vi "Periodic Tasks.vi"(8 "error in":errorcluster) -> ()   [LabVIEW 2018]
doc: "This VI runs in parallel to other tasks. It can contain as many user-defined periodic loops as you need. These can carry out PID or other sorts of timed response."
uses:
  SwerveRotationCalibrate.ctl
  <vilib>/Rock Robotics/WPI/ThirdParty/Phoenix-LabVIEW/Motor Controller/Controls/CTRE_Phoenix_MotorControl_NeutralMode.ctl
  <vilib>/Rock Robotics/WPI/ThirdParty/Phoenix-LabVIEW/Motor Controller/Controls/CTRE_Phoenix_MotorControl_ControlMode.ctl
  <vilib>/Rock Robotics/WPI/ThirdParty/Phoenix-LabVIEW/Motor Controller/Controls/CTRE_Phoenix_MotorControl_FeedbackDevice.ctl
  HatchModes.ctl
  ElevBasePos.ctl
  ElevModes.ctl
  SequenceActions.ctl
  d8969dce-e83f-414b-ab1b-b6caec8a5545.vi
  a102eae3-c5ed-494b-96cc-72fbbd712b4d.vi
  <vilib>/Rock Robotics/WPI/Utilities/WPI_GetSetVariantRefNum.vi
  <vilib>/Rock Robotics/Network Tables/NT Read Boolean.vi
  Robot Global Data.vi
  <vilib>/Rock Robotics/Network Tables/NT Write Numeric Array.vi
  <vilib>/Rock Robotics/Network Tables/NT Write String.vi
  <vilib>/Rock Robotics/Network Tables/NT Write Number.vi
  <vilib>/Rock Robotics/Network Tables/NT Write Boolean.vi
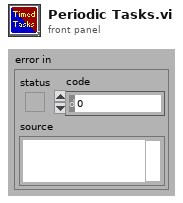
[diagram p1: front panel]
types:
  T1 = typedef "HatchModes.ctl" = enum16{"Travel", "PickPlace"}
  T2 = typedef "SwerveRotationCalibrate.ctl" = enum16{"Calibrate", "Home", "ManualHome", "ResetQuad", "Drive"}
  T3 = typedef "CTRE_Phoenix_MotorControl_NeutralMode.ctl" = enum8{"EEPROMSetting", "Override to Coast", "Override to Brake"}
  T4 = typedef "CTRE_Phoenix_MotorControl_ControlMode.ctl" = u16
  T5 = typedef "CTRE_Phoenix_MotorControl_FeedbackDevice.ctl" = i8
  T6 = cluster{"T0":u32, "Mode":T2, "Rotation Neutral Mode":T3, "Rotation Control Mode":T4, "Feedback Device":T5}
  T7 = cluster{"Yaw":dbl, "Roll":dbl, "Pitch":dbl, "Heading":dbl, "Fused Heading":dbl}
  T8 = typedef "ElevBasePos.ctl" = enum16{"NoChange", "Hatch", "Unused", "Carry", "Cargo"}
  T9 = typedef "WPI_JoystickDevRef.ctl" = cluster{"Device":T10}
  T10 = typedef "WPI_JoystickDeviceEnum.ctl" = enum16{"USB 0", "USB 1", "USB 2", "USB 3", "USB 4", "USB 5"}
  T11 = typedef "ElevModes.ctl" = enum16{"Manual", "Auto"}
  T12 = typedef "SequenceActions.ctl" = enum16{"HatchLatch", "MoveElev", "Ready"}
  T13 = typedef "WPI_DriverStationRobotMode2.ctl" = enum16{"Autonomous Disabled", "Autonomous Enabled", "Teleop Disabled", "Teleop Enabled", "Disconnected", "Finish", "Test Disabled", "Test Enabled", "Emergency Stopped"}
  T14 = cluster{"Buttons[0]":bool, "Buttons[1]":bool, "Buttons[2]":bool, "Buttons[3]":bool, "Buttons[4]":bool, "Buttons[5]":bool, "Buttons[6]":bool, "Buttons[7]":bool, "Buttons[8]":bool, "Buttons[9]":bool, "Buttons[10]":bool, "Buttons[11]":bool, "Buttons[12]":bool}
  T15 = cluster{"Motor1":cluster{"P":dbl, "I":dbl, "D":dbl}, "Motor3":cluster{"P":dbl, "I":dbl, "D":dbl}, "Motor2":cluster{"P":dbl, "I":dbl, "D":dbl}, "Motor4":cluster{"P":dbl, "I":dbl, "D":dbl}}
  T16 = typedef "WPI_CompressorDevRef.ctl" = cluster{"DevStatus":errorcluster, "Pneumatics Control Module":u8}
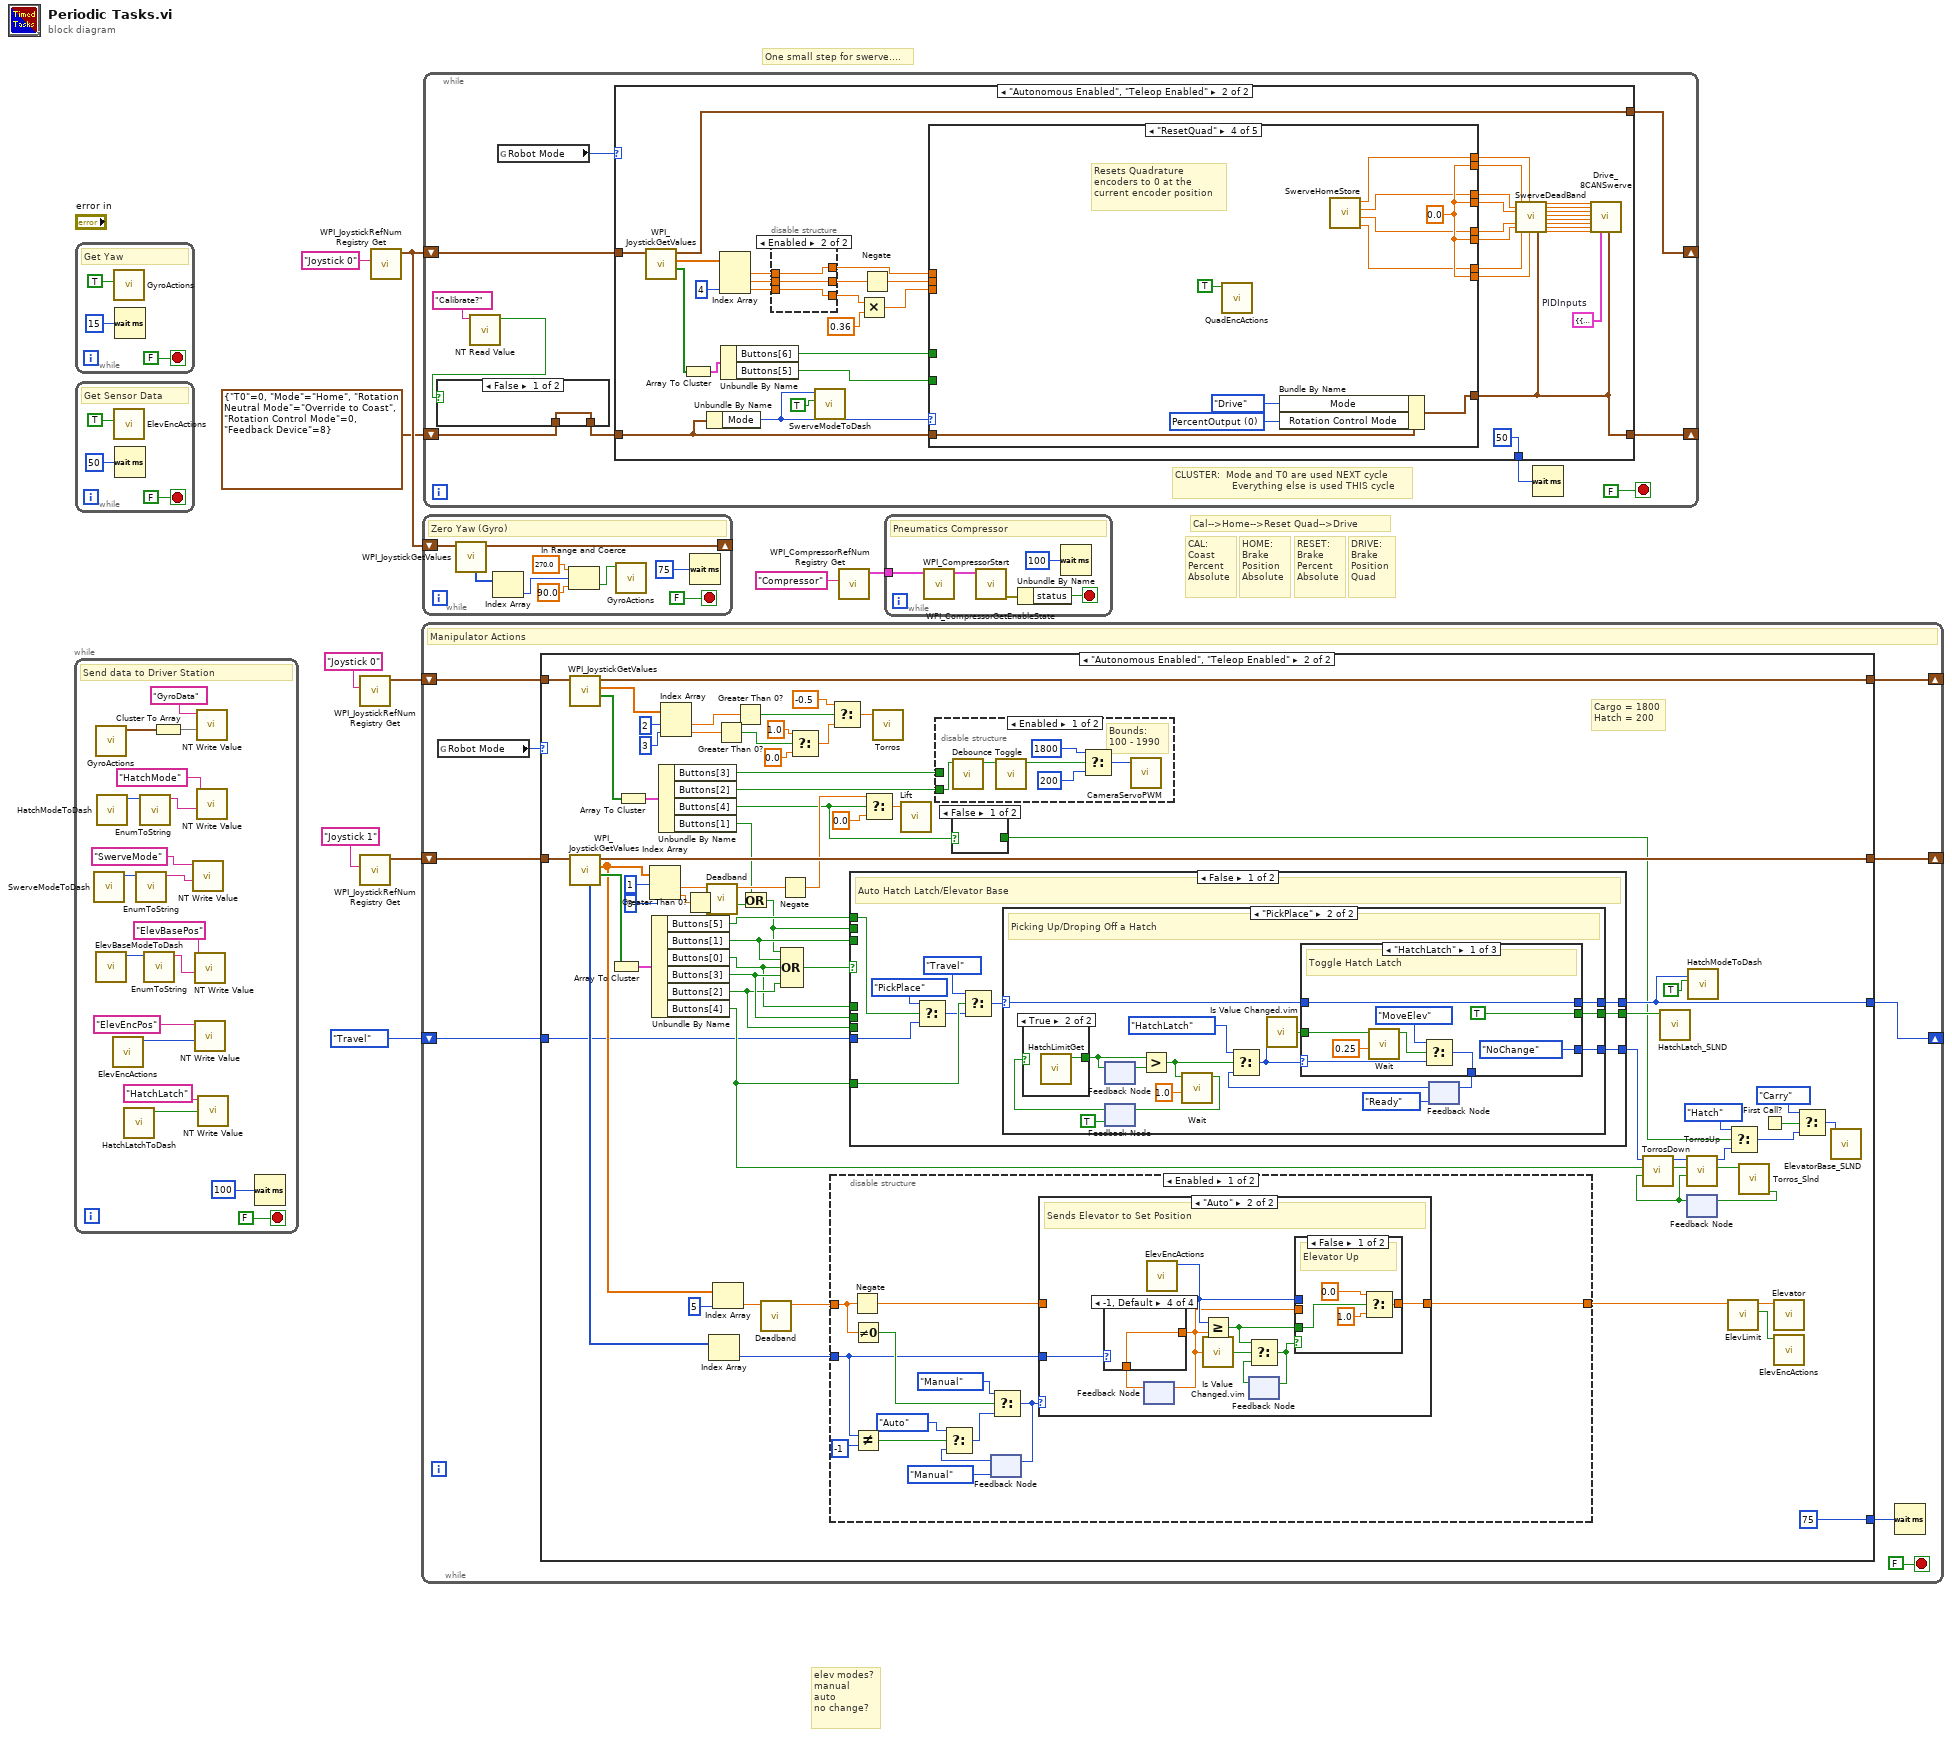
[diagram p0: block diagram]
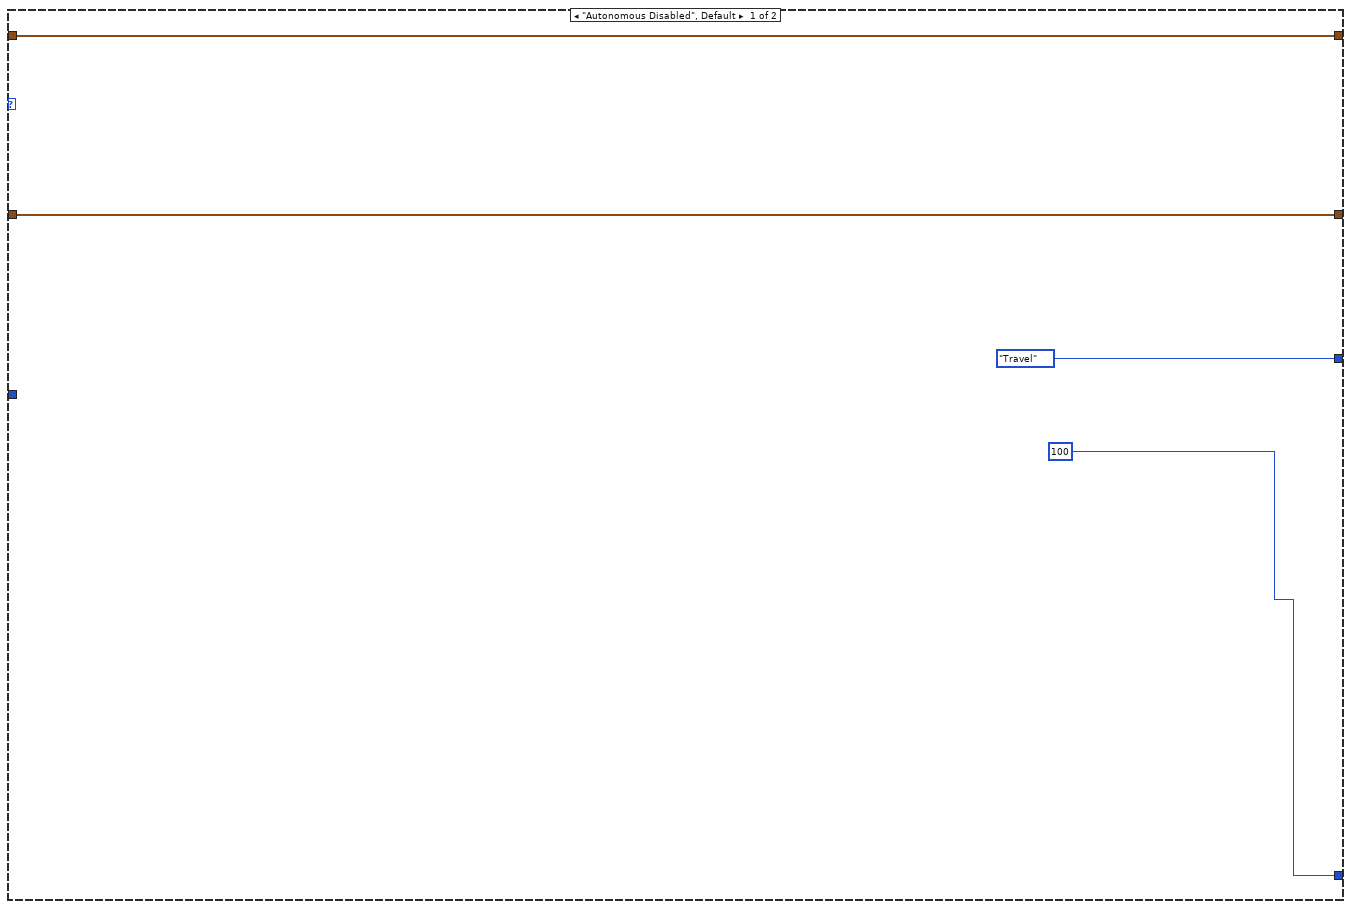
[diagram p2: hidden frame]
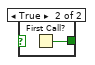
[diagram p3: hidden frame]
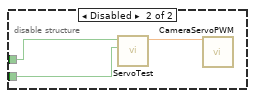
[diagram p4: hidden frame]
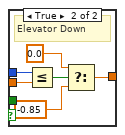
[diagram p6: hidden frame]
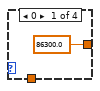
[diagram p7: hidden frame]
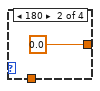
[diagram p8: hidden frame]
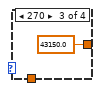
[diagram p9: hidden frame]
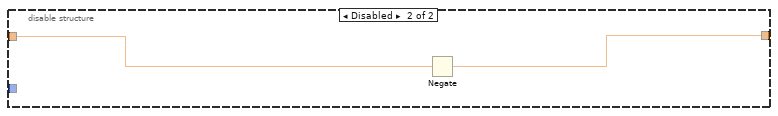
[diagram p10: hidden frame]
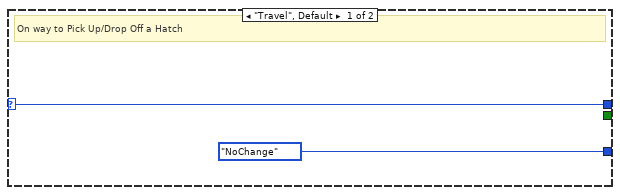
[diagram p11: hidden frame]
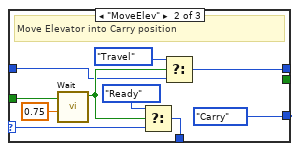
[diagram p13: hidden frame]
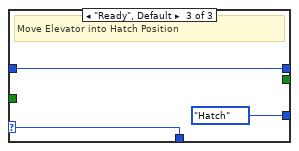
[diagram p14: hidden frame]
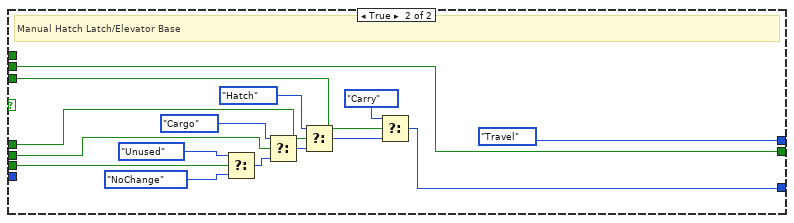
[diagram p15: hidden frame]
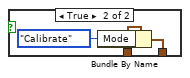
[diagram p16: hidden frame]
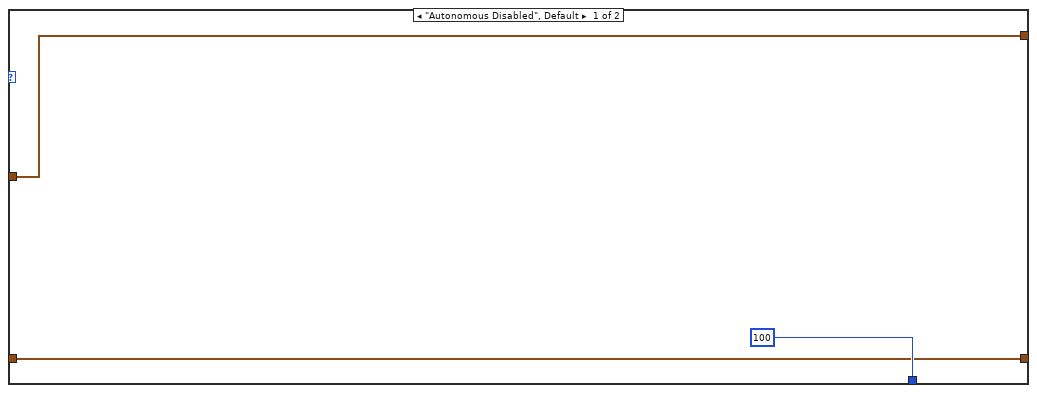
[diagram p17: hidden frame]
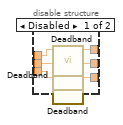
[diagram p18: hidden frame]
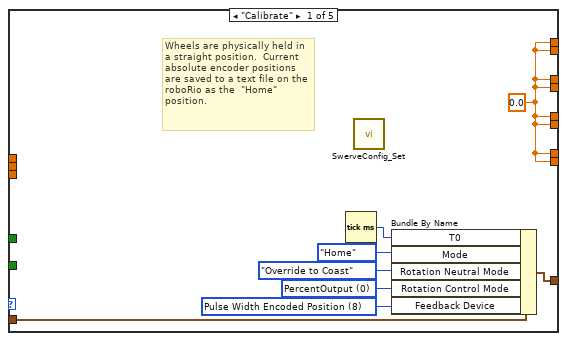
[diagram p19: hidden frame]
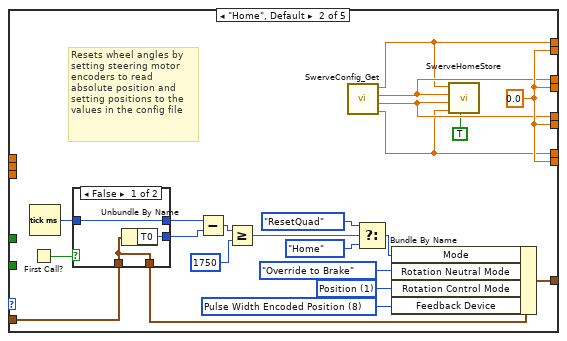
[diagram p20: hidden frame]
diagram:
  # "elev modes?\nmanual\nauto\nno change?"
  # "One small step for swerve...."
  # "DRIVE:\nBrake\nPosition\nQuad"
  # "RESET:\nBrake\nPercent\nAbsolute"
  # "HOME:\nBrake\nPosition\nAbsolute"
  # "Cal-->Home-->Reset Quad-->Drive"
  # "CAL:\nCoast\nPercent\nAbsolute"
  n1 = while {
    stop <- FALSE stop-if-true
    # "Send data to Driver Station"
    n2 = call "SwerveModeToDash.vi"() -> ("SwerveModeOut"=w18:T2)  [unwired: 11 in]
    n3 = call "GyroActions.vi"() -> ("YRPHfH"=w27:T7)  [unwired: 10 in, 1 out]
    n4 = call "ElevBaseModeToDash.vi"() -> ("ElevBasePosOut"=w13:T8)  [unwired: 11 in]
    n5 = call "HatchModeToDash.vi"() -> ("HatchModeOut"=w21:T1)  [unwired: 11 in]
    n6 = call "ElevEncActions.vi"() -> ("ElevEncPos"=w15:i32)  [unwired: 11 in]
    n7 = call "HatchLatchToDash.vi"() -> ("HatchLatchOut"=w11:bool)  [unwired: 11 in]
    n8 = call "EnumToString.vi"("Enum"=w18) -> ("String"=w17:string)  [unwired: 10 in]
    n9 = call "EnumToString.vi"("Enum"=w21) -> ("String"=w20:string)  [unwired: 10 in]
    n10 = call "EnumToString.vi"("Enum"=w13) -> ("String"=w22:string)  [unwired: 10 in]
    n11 = Cluster To Array(cluster=w27) -> (array=w26:dbl[])
    n12 = call-poly <vilib>:"NT Write Value.vi"("String"=w17, "Name"="SwerveMode") -> ()  [unwired: 9 in, 1 out]
    n13 = call-poly <vilib>:"NT Write Value.vi"("String"=w22, "Name"="ElevBasePos") -> ()  [unwired: 9 in, 1 out]
    n14 = call-poly <vilib>:"NT Write Value.vi"("Numeric"=w15, "Name"="ElevEncPos") -> ()  [unwired: 9 in, 1 out]
    n15 = call-poly <vilib>:"NT Write Value.vi"("Numeric Array"=w26, "Name"="GyroData") -> ()  [unwired: 9 in, 1 out]
    n16 = call-poly <vilib>:"NT Write Value.vi"("String"=w20, "Name"="HatchMode") -> ()  [unwired: 9 in, 1 out]
    n17 = call-poly <vilib>:"NT Write Value.vi"("Boolean"=w11, "Name"="HatchLatch") -> ()  [unwired: 9 in, 1 out]
    n18 = Wait (ms)(milliseconds to wait=u32 100 ("millisecond timer value")) -> ()  [unwired: 1 out]
  }
  n19 = while {
    stop <- FALSE stop-if-true
    # "Get Yaw"
    n20 = call "GyroActions.vi"("Update?"=TRUE ("Zero")) -> ()  [unwired: 9 in, 2 out]
    n21 = Wait (ms)(milliseconds to wait=u32 15) -> ()  [unwired: 1 out]
  }
  n22 = while {
    stop <- FALSE stop-if-true
    # "Get Sensor Data"
    n23 = call "ElevEncActions.vi"("Update?"=TRUE ("Zero")) -> ()  [unwired: 10 in, 1 out]
    n24 = Wait (ms)(milliseconds to wait=u32 50) -> ()  [unwired: 1 out]
  }
  n25 = call <vilib>:"WPI_JoystickRefNum Registry Get.vi"("refnum name"="Joystick 0") -> ("JoystickDevRef"=w2:T9)  [unwired: 1 in, 9 out]
  n26 = call <vilib>:"WPI_JoystickRefNum Registry Get.vi"("refnum name"="Joystick 1") -> ("JoystickDevRef"=w6:T9)  [unwired: 1 in, 9 out]
  n27 = call <vilib>:"WPI_JoystickRefNum Registry Get.vi"("refnum name"="Joystick 0") -> ("JoystickDevRef"=w9:T9)  [unwired: 1 in, 9 out]
  n28 = while {
    shift-right: [w37] -> _
    shift-left: HatchModes."Travel" -> [w38]
    shift-right: [w36] -> _
    shift-left: w6 -> [w42]
    shift-right: [w35] -> _
    shift-left: w2 -> [w39]
    stop <- FALSE stop-if-true
    # "Manipulator Actions"
    n29 = global read "Robot Global Data.vi" "Robot Mode"() -> (w43:T13)
    n30 = case shown="\"Autonomous Enabled\", \"Teleop Enabled\"" w43 {
      tunnel: w42 -> [w45 w114]
      tunnel: [u32 100 ("milliseconds to wait") u32 75 ("milliseconds to wait")] -> w40
      tunnel: w39 -> [w44 w108]
      tunnel: w38 -> [_ w61]
      tunnel: [HatchModes."Travel" w76] -> w37
      tunnel: [w45 w71] -> w36
      tunnel: [w44 w70] -> w35
      frame "Autonomous Disabled", Default {
      }
      frame "Autonomous Enabled", "Teleop Enabled" {
        # "Cargo = 1800\nHatch = 200"
        n31 = call <vilib>:"WPI_JoystickGetValues.vi"("JoystickDevRef"=w108) -> ("Buttons"=w109:bool[], "Axes"=w98:dbl[], "JoystickDevRef"=w70:T9)  [unwired: 6 in, 2 out]
        n32 = call <vilib>:"WPI_JoystickGetValues.vi"("JoystickDevRef"=w114) -> ("Buttons"=w113:bool[], "Axes"=w72:dbl[], "JoystickDevRef"=w71:T9, "POVs"=w111:i16[])  [unwired: 6 in, 1 out]
        n33 = Array To Cluster(array=w113) -> (cluster=w115:T14)
        n34 = Array To Cluster(array=w109) -> (cluster=w110:T14)
        n35 = Index Array(array=w72, index #1=1 ("index"), index #2=3 ("index")) -> (element #1=w69:dbl, element #2=w57:dbl)
        n36 = Unbundle By Name(w115) -> ("Buttons[5]"=w84:bool, "Buttons[1]"=w106:bool, "Buttons[0]"=w74:bool, "Buttons[3]"=w105:bool, "Buttons[2]"=w104:bool, "Buttons[4]"=w62:bool)
        n37 = Unbundle By Name(w110) -> ("Buttons[3]"=w59:bool, "Buttons[2]"=w60:bool, "Buttons[4]"=w51:bool, "Buttons[1]"=w55:bool)
        n38 = Index Array(array=w98, index #1=2 ("index"), index #2=3 ("index")) -> (element #1=w94:dbl, element #2=w95:dbl)
        n39 = Greater Than 0?(x=w57) -> (x > 0?=w56:bool)
        n40 = call "Deadband.vi"("Input"=w69) -> ("Output"=w66:dbl)  [unwired: 6 in]
        n41 = Index Array(array=w111) -> (element=w100:i16)  [unwired: 1 in]
        n42 = Index Array(array=w72, index=5) -> (element=w85:dbl)
        n43 = Greater Than 0?(x=w95) -> (x > 0?=w92:bool)
        n44 = Greater Than 0?(x=w94) -> (x > 0?=w93:bool)
        n45 = Or(x=w55, y=w56) -> (x .or. y?=w54:bool)
        n46 = call "Deadband.vi"("Input"=w85) -> ("Output"=w102:dbl)  [unwired: 6 in]
        n47 = Negate(x=w66) -> (-x=w67:dbl)
        n48 = Compound Arithmetic op=OR(w54, w106, w74, w105, w104) -> (w107:bool)
        n49 = Select(t=1.0, s=w92, f=0.0) -> (s? t:f=w91:dbl)
        n50 = disable-structure shown="Enabled" {
          disable-tunnel: w102 -> [w138 w164]
          disable-tunnel: [w137 w163] -> w101
          disable-tunnel: w100 -> [w126 _]
          frame Enabled {
            n51 = Negate(x=w138) -> (-x=w127:dbl)
            n52 = Not Equal To 0?(x=w138) -> (x != 0?=w131:bool)
            n53 = Not Equal?(x=w126, y=i16 -1) -> (x != y?=w129:bool)
            n54 = feedback #1(ElevModes."Manual") -> (w132:T11)
            n55 = Select(t=ElevModes."Auto", s=w129, f=w132) -> (s? t:f=w135:T11)
            n56 = Select(t=ElevModes."Manual", s=w131, f=w135) -> (s? t:f=w128:T11)
            n57 = feedback-in #1(w128) -> ()
            n58 = case shown="\"Auto\"" w128 {
              tunnel: w126 -> [_ w148]
              tunnel: [w139 w147] -> w137
              tunnel: w127 -> [w139 _]
              frame "Manual", Default {
                # "Uses Joystick Input"
              }
              frame "Auto" {
                # "Sends Elevator to Set Position"
                n59 = feedback #2() -> (w141:dbl)  [unwired: 1 in]
                n60 = case shown="-1, Default" w148 {
                  tunnel: [86300.0 ("Target") 0.0 ("Target") 43150.0 ("Target") w162] -> w140
                  tunnel: w141 -> [_ _ _ w162]
                  frame 0 {
                  }
                  frame 180 {
                  }
                  frame 270 {
                  }
                  frame -1, Default {
                  }
                }
                n61 = feedback-in #2(w140) -> ()
                n62 = call "ElevEncActions.vi"() -> ("ElevEncPos"=w142:i32)  [unwired: 11 in]
                n63 = Greater Or Equal?(x=w142, y=w140) -> (x >= y?=w143:bool)
                n64 = call "Is Value Changed.vim"("value"=w140) -> ("changed or first call?"=w146:bool)
                n65 = feedback #3() -> (w145:bool)  [unwired: 1 in]
                n66 = Select(t=w143, s=w146, f=w145) -> (s? t:f=w144:bool)
                n67 = feedback-in #3(w144) -> ()
                n68 = case shown="False" w144 {
                  tunnel: [w150 w154] -> w147
                  tunnel: w140 -> [_ w156]
                  tunnel: w142 -> [_ w153]
                  tunnel: w143 -> [w149 _]
                  frame False {
                    # "Elevator Up"
                    n69 = Select(t=0.0, s=w149, f=1.0) -> (s? t:f=w150:dbl)
                  }
                  frame True {
                    # "Elevator Down"
                    n70 = Less Or Equal?(x=w153, y=w156) -> (x <= y?=w155:bool)
                    n71 = Select(t=0.0, s=w155, f=-0.85) -> (s? t:f=w154:dbl)
                  }
                }
              }
            }
          }
          frame Disabled {
            n72 = Negate(x=w164) -> (-x=w163:dbl)
          }
        }
        n73 = Select(t=-0.5, s=w93, f=w91) -> (s? t:f=w90:dbl)
        n74 = case shown="False" w107 {
          tunnel: w61 -> [w169 _]
          tunnel: [w174 HatchModes."Travel"] -> w76
          tunnel: [w173 w230] -> w103
          tunnel: w54 -> [_ w230]
          tunnel: w106 -> [_ w229]
          tunnel: w74 -> [_ w228]
          tunnel: w105 -> [_ w227]
          tunnel: w104 -> [_ w226]
          tunnel: w84 -> [w171 _]
          tunnel: [w170 w217] -> w81
          tunnel: w62 -> [w168 _]
          frame False {
            # "Auto Hatch Latch/Elevator Base"
            n75 = Select(t=HatchModes."PickPlace", s=w171, f=w169) -> (s? t:f=w166:T1)
            n76 = Select(t=HatchModes."Travel", s=w168, f=w166) -> (s? t:f=w165:T1)
            n77 = case shown="\"PickPlace\"" w165 {
              selector: w165 -> [w176 w193]
              tunnel: [w176 w192] -> w174
              tunnel: [_ w191] -> w173
              tunnel: [ElevBasePos."NoChange" w184] -> w170
              frame "Travel", Default {
                # "On way to Pick Up/Drop Off a Hatch"
              }
              frame "PickPlace" {
                # "Picking Up/Droping Off a Hatch"
                n78 = feedback #4() -> (w179:bool)  [unwired: 1 in]
                n79 = feedback #5(TRUE ("Completed")) -> (w181:bool)
                n80 = case shown="True" w181 {
                  tunnel: [_ w194] -> w177
                  frame False {
                  }
                  frame True {
                    n81 = call "HatchLimitGet.vi"() -> ("Pressed?"=w194:bool)  [unwired: 11 in]
                  }
                }
                n82 = feedback-in #4(w177) -> ()
                n83 = Greater?(x=w177, y=w179) -> (0:w178:bool)
                n84 = call "Wait.vi"("Target Time (s)"=1.0, "Start Timer?"=w178) -> ("Completed"=w182:bool)  [unwired: 8 in, 1 out]
                n85 = feedback-in #5(w182) -> ()
                n86 = feedback #6(SequenceActions."Ready" ("SequenceAction")) -> (w188:T12)
                n87 = Select(t=SequenceActions."HatchLatch" ("SequenceAction"), s=w178, f=w188) -> (s? t:f=w190:T12)
                n88 = call "Is Value Changed.vim"("value"=w190) -> ("changed or first call?"=w185:bool)
                n89 = case shown="\"HatchLatch\"" w190 {
                  selector: w190 -> [w202 w213 w215]
                  tunnel: [w201 w212 w215] -> w189
                  tunnel: w193 -> [w200 w209 w216]
                  tunnel: [w200 w208 w216] -> w192
                  tunnel: [TRUE _ _] -> w191
                  tunnel: w185 -> [w197 w206 _]
                  tunnel: [ElevBasePos."NoChange" ElevBasePos."Carry" ElevBasePos."Hatch"] -> w184
                  frame "HatchLatch" {
                    # "Toggle Hatch Latch"
                    n90 = call "Wait.vi"("Target Time (s)"=0.25, "Start Timer?"=w197) -> ("Completed"=w203:bool)  [unwired: 8 in, 1 out]
                    n91 = Select(t=SequenceActions."MoveElev" ("SequenceAction"), s=w203, f=w202) -> (s? t:f=w201:T12)
                  }
                  frame "MoveElev" {
                    # "Move Elevator into Carry position"
                    n92 = call "Wait.vi"("Target Time (s)"=0.75, "Start Timer?"=w206) -> ("Completed"=w211:bool)  [unwired: 8 in, 1 out]
                    n93 = Select(t=SequenceActions."Ready" ("SequenceAction"), s=w211, f=w213) -> (s? t:f=w212:T12)
                    n94 = Select(t=HatchModes."Travel", s=w211, f=w209) -> (s? t:f=w208:T1)
                  }
                  frame "Ready", Default {
                    # "Move Elevator into Hatch Position"
                  }
                }
                n95 = feedback-in #6(w189) -> ()
              }
            }
          }
          frame True {
            # "Manual Hatch Latch/Elevator Base"
            n96 = Select(t=ElevBasePos."Unused", s=w226, f=ElevBasePos."NoChange") -> (s? t:f=w225:T8)
            n97 = Select(t=ElevBasePos."Cargo", s=w227, f=w225) -> (s? t:f=w224:T8)
            n98 = Select(t=ElevBasePos."Hatch", s=w228, f=w224) -> (s? t:f=w223:T8)
            n99 = Select(t=ElevBasePos."Carry", s=w229, f=w223) -> (s? t:f=w217:T8)
          }
        }
        n100 = Select(t=w67, s=w51, f=0.0 ("t")) -> (s? t:f=w53:dbl)
        n101 = call "Torros.vi"("Power"=w90) -> ()  [unwired: 11 in]
        n102 = call "Lift.vi"("Power"=w53) -> ()  [unwired: 11 in]
        n103 = disable-structure shown="Enabled" {
          disable-tunnel: w60 -> [w118 w125]
          disable-tunnel: w59 -> [_ w124]
          frame Enabled {
            # "Bounds: 100 - 1990"
            n104 = call "Debounce.vi"("booleanIn"=w118) -> ("booleanOut"=w119:bool)  [unwired: 10 in]
            n105 = call "Toggle.vi"("booleanIn"=w119) -> ("booleanOut"=w120:bool)  [unwired: 10 in]
            n106 = Select(t=1800, s=w120, f=200) -> (s? t:f=w117:i32)
            n107 = call "CameraServoPWM.vi"("Position"=w117) -> ()  [unwired: 11 in]
          }
          frame Disabled {
            n108 = call "ServoTest.vi"("Down"=w125, "Up"=w124) -> ("Angle"=w123:dbl)  [unwired: 9 in]
            n109 = call "CameraServoPWM.vi"("Position"=w123) -> ()  [unwired: 11 in]
          }
        }
        n110 = case shown="False" w51 {
          tunnel: [_ w116] -> w50
          frame False {
          }
          frame True {
            n111 = First Call?() -> (First Call?: T/F=w116:bool)
          }
        }
        n112 = call "HatchLatch_SLND.vi"("Toggle?"=w103) -> ()  [unwired: 11 in]
        n113 = feedback #7() -> (w79:bool)  [unwired: 1 in]
        n114 = call "TorrosDown.vi"("TorrosCurrPos"=w79, "TorrosButton"=w62, "ElevBasePosIn"=w81) -> ("TorrosOut"=w82:bool, "ElevBasePosOut"=w80:T8)  [unwired: 7 in]
        n115 = call "TorrosUp.vi"("TorrosCurrPos"=w79, "TorrosIn"=w82, "ElevBasePosIn"=w80) -> ("TorrosOut"=w83:bool, "ElevBasePosOut"=w49:T8)  [unwired: 7 in]
        n116 = call "HatchModeToDash.vi"("Update?"=TRUE, "HatchModeIn"=w76) -> ()  [unwired: 9 in, 1 out]
        n117 = call "ElevLimit.vi"("PowerIn"=w101) -> ("BotLimit"=w75:bool, "PowerOut"=w99:dbl)  [unwired: 8 in, 1 out]
        n118 = Select(t=ElevBasePos."Hatch", s=w50, f=w49) -> (s? t:f=w48:T8)
        n119 = call "Torros_Slnd.vi"("Toggle?"=w83) -> ("CurrState"=w78:bool)  [unwired: 10 in]
        n120 = feedback-in #7(w78) -> ()
        n121 = First Call?() -> (First Call?: T/F=w64:bool)
        n122 = call "Elevator.vi"("Power"=w99) -> ()  [unwired: 11 in]
        n123 = call "ElevEncActions.vi"("Zero?"=w75) -> ()  [unwired: 10 in, 1 out]
        n124 = Select(t=ElevBasePos."Carry", s=w64, f=w48) -> (s? t:f=w65:T8)
        n125 = call "ElevatorBase_SLND.vi"("ElevBasePosIn"=w65) -> ()  [unwired: 11 in]
      }
    }
    n126 = Wait (ms)(milliseconds to wait=w40) -> ()  [unwired: 1 out]
  }
  n127 = while {
    shift-right: [w233] -> _
    shift-left: w9 -> [w240]
    stop <- FALSE stop-if-true
    # "Zero Yaw (Gyro)"
    n128 = call <vilib>:"WPI_JoystickGetValues.vi"("JoystickDevRef"=w240) -> ("JoystickDevRef"=w233:T9, "POVs"=w238:i16[])  [unwired: 6 in, 3 out]
    n129 = Index Array(array=w238) -> (element=w237:i16)  [unwired: 1 in]
    n130 = In Range and Coerce(upper limit=270.0, x=w237, lower limit=90.0) -> (In Range?=w236:bool)  [unwired: 1 out]
    n131 = call "GyroActions.vi"("Zero"=w236) -> ()  [unwired: 9 in, 2 out]
    n132 = Wait (ms)(milliseconds to wait=u32 75) -> ()  [unwired: 1 out]
  }
  n133 = while {
    shift-right: [w248] -> _
    shift-left: w9 -> [w249]
    shift-right: [w247] -> _
    shift-left: T6 {"T0"=0, "Mode"=enum."Home", "Rotation Neutral Mode"=enum."Override to Coast", "Rotation Control Mode"=0, "Feedback Device"=8} ("RotationSettings") -> [w243]
    stop <- FALSE stop-if-true
    # "CLUSTER:  Mode and T0 are used NEXT cycle\n                   Everything else is used THIS cycle"
    n134 = call-poly <vilib>:"NT Read Value.vi"("Name"="Calibrate?") -> ("Boolean"=w241:bool)  [unwired: 9 in, 1 out]
    n135 = case shown="False" w241 {
      tunnel: w243 -> [w251 w254]
      tunnel: [w251 w253] -> w242
      frame False {
      }
      frame True {
        n136 = Bundle By Name(cluster=w254, "Mode"=SwerveRotationCalibrate."Calibrate") -> (w253:T6)
      }
    }
    n137 = global read "Robot Global Data.vi" "Robot Mode"() -> (w245:T13)
    n138 = case shown="\"Autonomous Enabled\", \"Teleop Enabled\"" w245 {
      tunnel: w249 -> [w255 w296]
      tunnel: [w255 w295] -> w248
      tunnel: [w256 w268] -> w247
      tunnel: w242 -> [w256 w289]
      tunnel: [u32 100 ("milliseconds to wait") u32 50 ("milliseconds to wait")] -> w246
      frame "Autonomous Disabled", Default {
      }
      frame "Autonomous Enabled", "Teleop Enabled" {
        w290 = T15 {"Motor1"={"P"=4.0, "I"=0.0, "D"=64.0}, "Motor3"={"P"=4.0, "I"=0.0, "D"=64.0}, "Motor2"={"P"=4.0, "I"=0.0, "D"=64.0}, "Motor4"={"P"=4.0, "I"=0.0, "D"=64.0}}  # PIDInputs
        n139 = call <vilib>:"WPI_JoystickGetValues.vi"("JoystickDevRef"=w296) -> ("Buttons"=w293:bool[], "Axes"=w294:dbl[], "JoystickDevRef"=w295:T9)  [unwired: 6 in, 2 out]
        n140 = Array To Cluster(array=w293) -> (cluster=w292:T14)
        n141 = Unbundle By Name(w289) -> ("Mode"=w262:T2)
        n142 = Index Array(array=w294, index #3=4 ("index")) -> (element #1=w291:dbl, element #2=w267:dbl, element #3=w259:dbl)  [unwired: 2 in]
        n143 = Unbundle By Name(w292) -> ("Buttons[6]"=w258:bool, "Buttons[5]"=w263:bool)
        n144 = disable-structure shown="Enabled" {
          disable-tunnel: w259 -> [w302 w303]
          disable-tunnel: w291 -> [w301 w305]
          disable-tunnel: [w300 w304] -> w287
          disable-tunnel: [w299 w305] -> w285
          disable-tunnel: w267 -> [w298 w304]
          disable-tunnel: [w297 w303] -> w264
          frame Disabled {
            n145 = call "Deadband.vi"("Input"=w301) -> ("Output"=w299:dbl)  [unwired: 6 in]
            n146 = call "Deadband.vi"("Input"=w298) -> ("Output"=w300:dbl)  [unwired: 6 in]
            n147 = call "Deadband.vi"("Input"=w302) -> ("Output"=w297:dbl)  [unwired: 6 in]
          }
          frame Enabled {
          }
        }
        n148 = call "SwerveModeToDash.vi"("Update?"=TRUE, "SwerveModeIn"=w262) -> ()  [unwired: 9 in, 1 out]
        n149 = Multiply(x=w264, y=0.36) -> (x*y=w266:dbl)
        n150 = Negate(x=w287) -> (-x=w286:dbl)
        n151 = case shown="\"ResetQuad\"" w262 {
          tunnel: [w307 w335 w360 w372 w408] -> w281
          tunnel: [w307 w315 w342 w367 w402] -> w284
          tunnel: [w307 w335 w360 w372 w406] -> w283
          tunnel: [w307 w318 w342 w368 w407] -> w282
          tunnel: [w307 w335 w360 w372 w412] -> w277
          tunnel: [w307 w316 w342 w370 w411] -> w278
          tunnel: [w307 w335 w360 w372 w410] -> w280
          tunnel: [w307 w317 w342 w369 w409] -> w279
          tunnel: w289 -> [w313 w320 w345 w376 w399]
          tunnel: [w311 w331 w356 w375 w397] -> w268
          tunnel: w263 -> [_ _ _ _ w394]
          tunnel: w286 -> [_ _ _ _ w390]
          tunnel: w266 -> [_ _ _ _ w389]
          tunnel: w285 -> [_ _ _ _ w388]
          tunnel: w258 -> [_ _ _ _ w378]
          frame "Calibrate" {
            w307 = 0.0 ("P")
            w310 = T4 0 items=["PercentOutput"=0, "Position"=1, "Velocity"=2, "Current"=3, "Follower"=5, "MotionProfile"=6, "MotionMagic"=7, "MotionProfileArc"=10, "Disabled"=15] ("Rotation Control Mode")
            w312 = T5 8 items=["None"=-1, "QuadEncoder"=0, "Analog"=2, "Tachometer"=4, "Pulse Width Encoded Position"=8, "Sensor Sum (S0 + S1)"=9, "Sensor Difference (D0 - D1)"=10, "Remote Source 0"=11, "Remote Source 1"=12, "Software Emulated"=15] ("Feedback Device")
            # "Wheels are physically held in a straight position.  Current absolute encoder positions are saved to a text file on the roboRio as the  \"Home\" position."
            n152 = Tick Count (ms)() -> (millisecond timer value=w306:u32)
            n153 = call "SwerveConfig_Set.vi"() -> ()  [unwired: 12 in]
            n154 = Bundle By Name(cluster=w313, "T0"=w306, "Mode"=SwerveRotationCalibrate."Home", "Rotation Neutral Mode"=CTRE_Phoenix_MotorControl_NeutralMode."Override to Coast", "Rotation Control Mode"=w310, "Feedback Device"=w312) -> (w311:T6)
          }
          frame "Home", Default {
            w333 = T4 1 items=["PercentOutput"=0, "Position"=1, "Velocity"=2, "Current"=3, "Follower"=5, "MotionProfile"=6, "MotionMagic"=7, "MotionProfileArc"=10, "Disabled"=15] ("Rotation Control Mode")
            w334 = T5 8 items=["None"=-1, "QuadEncoder"=0, "Analog"=2, "Tachometer"=4, "Pulse Width Encoded Position"=8, "Sensor Sum (S0 + S1)"=9, "Sensor Difference (D0 - D1)"=10, "Remote Source 0"=11, "Remote Source 1"=12, "Software Emulated"=15] ("Feedback Device")
            w335 = 0.0 ("P")
            # "Resets wheel angles by setting steering motor encoders to read absolute position and setting positions to the values in the config file"
            n155 = First Call?() -> (First Call?: T/F=w324:bool)
            n156 = Tick Count (ms)() -> (millisecond timer value=w323:u32)
            n157 = case shown="False" w324 {
              tunnel: w320 -> [w337 w341]
              tunnel: w323 -> [w338 w339]
              tunnel: [w338 w339] -> w322
              tunnel: [w337 w340] -> w321
              tunnel: [w336 w339] -> w319
              frame False {
                n158 = Unbundle By Name(w337) -> ("T0"=w336:u32)
              }
              frame True {
                n159 = Bundle By Name(cluster=w341, "T0"=w339) -> (w340:T6)
              }
            }
            n160 = Subtract(x=w322, y=w319) -> (x-y=w327:u32)
            n161 = Greater Or Equal?(x=w327, y=u32 1750) -> (x >= y?=w326:bool)
            n162 = call "SwerveConfig_Get.vi"() -> ("RearRightHome"=w316:dbl, "RearLeftHome"=w317:dbl, "FrontRightHome"=w318:dbl, "FrontLeftHome"=w315:dbl)  [unwired: 8 in]
            n163 = Select(t=SwerveRotationCalibrate."ResetQuad" ("Mode"), s=w326, f=SwerveRotationCalibrate."Home" ("Mode")) -> (s? t:f=w330:T2)
            n164 = Bundle By Name(cluster=w321, "Mode"=w330, "Rotation Neutral Mode"=CTRE_Phoenix_MotorControl_NeutralMode."Override to Brake", "Rotation Control Mode"=w333, "Feedback Device"=w334) -> (w331:T6)
            n165 = call "SwerveHomeStore.vi"("Update?"=TRUE, "RearRightHomeIn"=w316, "RearLeftHomeIn"=w317, "FrontRightHomeIn"=w318, "FrontLeftHomeIn"=w315) -> ()  [unwired: 3 in, 4 out]
          }
          frame "ManualHome" {
            w342 = 0.0 ("P")
            w358 = T4 1 items=["PercentOutput"=0, "Position"=1, "Velocity"=2, "Current"=3, "Follower"=5, "MotionProfile"=6, "MotionMagic"=7, "MotionProfileArc"=10, "Disabled"=15] ("Rotation Control Mode")
            w359 = T5 8 items=["None"=-1, "QuadEncoder"=0, "Analog"=2, "Tachometer"=4, "Pulse Width Encoded Position"=8, "Sensor Sum (S0 + S1)"=9, "Sensor Difference (D0 - D1)"=10, "Remote Source 0"=11, "Remote Source 1"=12, "Software Emulated"=15] ("Feedback Device")
            w360 = 0.0 ("P")
            # "Resets wheel angles by setting steering motor encoders to read absolute position and setting positions to the values in the config file"
            n166 = First Call?() -> (First Call?: T/F=w349:bool)
            n167 = Tick Count (ms)() -> (millisecond timer value=w348:u32)
            n168 = case shown="False" w349 {
              tunnel: w345 -> [w362 w366]
              tunnel: w348 -> [w363 w364]
              tunnel: [w363 w364] -> w347
              tunnel: [w362 w365] -> w346
              tunnel: [w361 w364] -> w344
              frame False {
                n169 = Unbundle By Name(w362) -> ("T0"=w361:u32)
              }
              frame True {
                n170 = Bundle By Name(cluster=w366, "T0"=w364) -> (w365:T6)
              }
            }
            n171 = Subtract(x=w347, y=w344) -> (x-y=w352:u32)
            n172 = Greater Or Equal?(x=w352, y=u32 1750) -> (x >= y?=w351:bool)
            n173 = Select(t=SwerveRotationCalibrate."ResetQuad" ("Mode"), s=w351, f=SwerveRotationCalibrate."ManualHome" ("Mode")) -> (s? t:f=w355:T2)
            n174 = Bundle By Name(cluster=w346, "Mode"=w355, "Rotation Neutral Mode"=CTRE_Phoenix_MotorControl_NeutralMode."Override to Brake", "Rotation Control Mode"=w358, "Feedback Device"=w359) -> (w356:T6)
            n175 = call "SwerveHomeStore.vi"("Update?"=TRUE, "RearRightHomeIn"=w342, "RearLeftHomeIn"=w342, "FrontRightHomeIn"=w342, "FrontLeftHomeIn"=w342) -> ()  [unwired: 3 in, 4 out]
          }
          frame "ResetQuad" {
            w373 = T4 0 items=["PercentOutput"=0, "Position"=1, "Velocity"=2, "Current"=3, "Follower"=5, "MotionProfile"=6, "MotionMagic"=7, "MotionProfileArc"=10, "Disabled"=15] ("Rotation Control Mode")
            w372 = 0.0 ("P")
            # "Resets Quadrature encoders to 0 at the current encoder position"
            n176 = call "QuadEncActions.vi"("Zero?"=TRUE ("Reset?")) -> ()  [unwired: 7 in, 4 out]
            n177 = Bundle By Name(cluster=w376, "Mode"=SwerveRotationCalibrate."Drive", "Rotation Control Mode"=w373) -> (w375:T6)
            n178 = call "SwerveHomeStore.vi"() -> ("RearRightHomeOut"=w370:dbl, "RearLeftHomeOut"=w369:dbl, "FrontRightHomeOut"=w368:dbl, "FrontLeftHomeOut"=w367:dbl)  [unwired: 8 in]
          }
          frame "Drive" {
            w396 = T4 1 items=["PercentOutput"=0, "Position"=1, "Velocity"=2, "Current"=3, "Follower"=5, "MotionProfile"=6, "MotionMagic"=7, "MotionProfileArc"=10, "Disabled"=15] ("Rotation Control Mode")
            w398 = T5 0 items=["None"=-1, "QuadEncoder"=0, "Analog"=2, "Tachometer"=4, "Pulse Width Encoded Position"=8, "Sensor Sum (S0 + S1)"=9, "Sensor Difference (D0 - D1)"=10, "Remote Source 0"=11, "Remote Source 1"=12, "Software Emulated"=15] ("Feedback Device")
            # "Creates a deadband for all axes and inverts y-axis so that pushing the stick forward gives a positive value"
            n179 = Select(t=SwerveRotationCalibrate."Home" ("Mode"), s=w394, f=SwerveRotationCalibrate."Drive" ("Mode")) -> (s? t:f=w380:T2)
            n180 = Select(t=SwerveRotationCalibrate."ManualHome" ("Mode"), s=w378, f=w380) -> (s? t:f=w379:T2)
            n181 = call "SwerveMath.vi"("X-Axis"=w388, "Y-Axis"=w390, "Turn"=w389) -> ("FrontLeftAngle"=w400:dbl, "FrontLeftDrive"=w387:dbl, "FrontRightAngle"=w386:dbl, "FrontRightDrive"=w385:dbl, "RearLeftAngle"=w384:dbl, "RearLeftDrive"=w383:dbl, "RearRightAngle"=w382:dbl, "RearRightDrive"=w381:dbl)  [unwired: 17 in]
            n182 = call "QuadEncActions.vi"() -> ("RearRightQuadPos"=w404:i32, "RearLeftQuadPos"=w403:i32, "FrontRightQuadPos"=w405:i32, "FrontLeftQuadPos"=w401:i32)  [unwired: 8 in]
            n183 = Tick Count (ms)() -> (millisecond timer value=w391:u32)
            n184 = Bundle By Name(cluster=w399, "T0"=w391, "Mode"=w379, "Rotation Neutral Mode"=CTRE_Phoenix_MotorControl_NeutralMode."Override to Brake", "Rotation Control Mode"=w396, "Feedback Device"=w398) -> (w397:T6)
            n185 = call "SwerveWheelHeadingCalc.vi"("DriveIn"=w387, "Target"=w400, "Current"=w401) -> ("DriveOut"=w406:dbl, "TargetFinal"=w402:dbl)  [unwired: 7 in]
            n186 = call "SwerveWheelHeadingCalc.vi"("DriveIn"=w385, "Target"=w386, "Current"=w405) -> ("DriveOut"=w408:dbl, "TargetFinal"=w407:dbl)  [unwired: 7 in]
            n187 = call "SwerveWheelHeadingCalc.vi"("DriveIn"=w383, "Target"=w384, "Current"=w403) -> ("DriveOut"=w410:dbl, "TargetFinal"=w409:dbl)  [unwired: 7 in]
            n188 = call "SwerveWheelHeadingCalc.vi"("DriveIn"=w381, "Target"=w382, "Current"=w404) -> ("DriveOut"=w412:dbl, "TargetFinal"=w411:dbl)  [unwired: 7 in]
          }
        }
        n189 = call "SwerveDeadBand.vi"("FrontRightRotationIn"=w282, "FrontRightDriveIn"=w281, "RearLeftRotationIn"=w279, "RearLeftDriveIn"=w280, "FrontLeftDriveIn"=w283, "RearRightRotationIn"=w278, "FrontLeftRotationIn"=w284, "RearRightDriveIn"=w277, "RotationSettings"=w268) -> ("FrontLeftRotationOut"=w276:dbl, "FrontLeftDriveOut"=w275:dbl, "FrontRightRotationOut"=w274:dbl, "FrontRightDriveOut"=w273:dbl, "RearLeftRotationOut"=w272:dbl, "RearLeftDriveOut"=w271:dbl, "RearRightRotationOut"=w270:dbl, "RearRightDriveOut"=w269:dbl)  [unwired: 11 in]
        n190 = call "Drive_8CANSwerve.vi"("FrontLeftRotation"=w276, "FrontLeftDrive"=w275, "FrontRightRotation"=w274, "FrontRightDrive"=w273, "RearLeftRotation"=w272, "RearLeftDrive"=w271, "RearRightRotation"=w270, "RearRightDrive"=w269, "PIDInputs"=w290, "RotationSettings"=w268) -> ()  [unwired: 18 in]
      }
    }
    n191 = Wait (ms)(milliseconds to wait=w246) -> ()  [unwired: 1 out]
  }
  n192 = call <vilib>:"WPI_CompressorRefNum Registry Get.vi"("refnum name"="Compressor") -> ("CompressorDevRef"=w4:T16)  [unwired: 9 in, 1 out]
  n193 = while {
    tunnel: w4 -> [w415]
    stop <- w416 stop-if-true
    # "Pneumatics Compressor"
    n194 = call <vilib>:"WPI_CompressorStart.vi"("CompressorDevRef"=w415) -> ("CompressorDevRef"=w414:T16)  [unwired: 9 in, 1 out]
    n195 = call <vilib>:"WPI_CompressorGetEnableState.vi"("CompressorDevRef"=w414) -> ("error out"=w413:errorcluster)  [unwired: 1 in, 9 out]
    n196 = Unbundle By Name(w413) -> ("status"=w416:bool)
    n197 = Wait (ms)(milliseconds to wait=u32 100) -> ()  [unwired: 1 out]
  }
